vi "04_DAC1curCompensation.vi"(9 "DAC1volt, V":dbl, 11 "DAC1curIN, mA":dbl) -> (1 "CurrentError":bool, 3 "DAC1curOUT, mA":dbl)   [LabVIEW 2017]
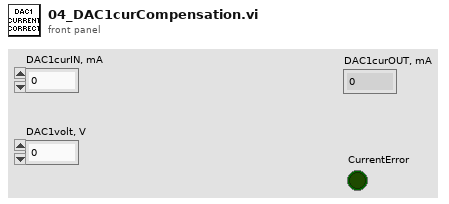
[diagram p1: front panel]
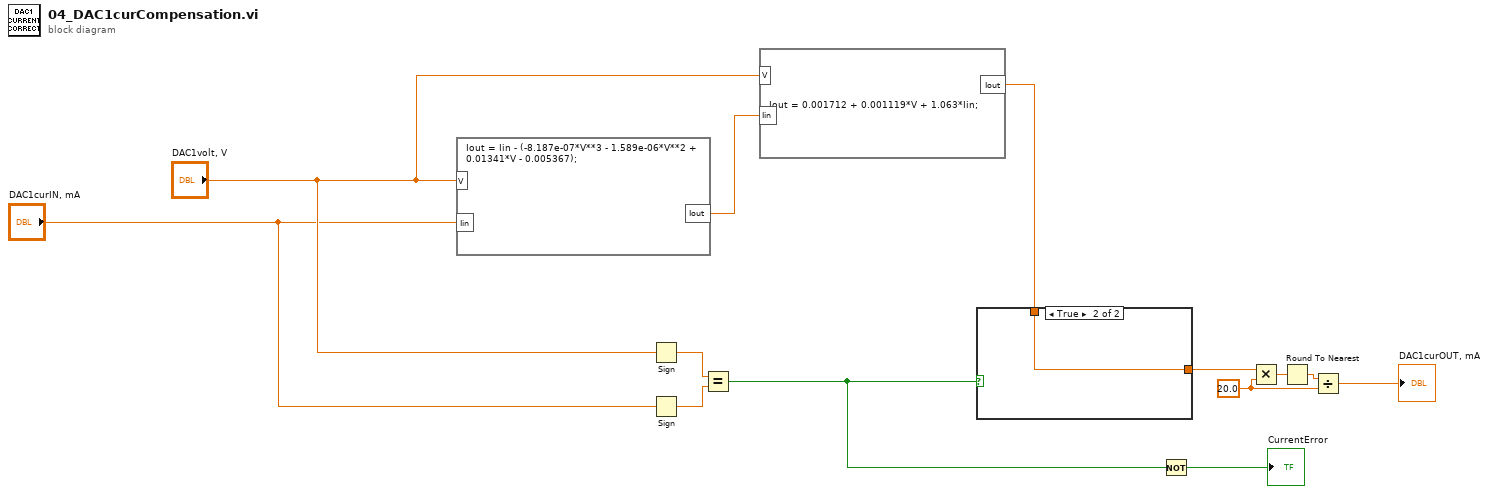
[diagram p0: block diagram]
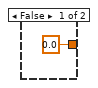
[diagram p2: hidden frame]
diagram:
  w13 = 20.0
  n1 = formula code="Iout = Iin - (-8.187e-07*V**3 - 1.589e-06*V**2 +  0.01341*V - 0.005367);"("V"="DAC1volt, V", "Iin"="DAC1curIN, mA") -> ("Iout"=w9:dbl)
  n2 = Sign(1:"DAC1volt, V") -> (0:w8:dbl)
  n3 = Sign(1:"DAC1curIN, mA") -> (0:w7:dbl)
  n4 = Equal?(x=w8, y=w7) -> (x = y?=w2:bool)
  n5 = formula code="Iout = 0.001712 + 0.001119*V + 1.063*Iin;"("V"="DAC1volt, V", "Iin"=w9) -> ("Iout"=w4:dbl)
  n6 = case shown="True" w2 {
    tunnel: w4 -> [_ w15]
    tunnel: [0.0 ("Iout") w15] -> w3
    frame False {
    }
    frame True {
    }
  }
  n7 = Not(x=w2) -> (.not. x?=→"CurrentError":bool)
  n8 = Multiply(x=w3, y=w13) -> (x*y=w12:dbl)
  n9 = Round To Nearest(number=w12) -> (nearest integer value=w11:dbl)
  n10 = Divide(x=w11, y=w13) -> (x/y=→"DAC1curOUT, mA":dbl)
